vi "earthquake and Tsunami version 2.vi"() -> ()   [LabVIEW 2019]
uses:
  <vilib>/imath/engines/lvmath2/RunTimeEngine/Managers/WorkSpace/UID Generator.vi
  <vilib>/imath/engines/lvmath2/RunTimeEngine/RunTimeType/NIMS_RunTimeType_From StrictType (excl LVString).vi
  <instcachedir>/0/NIMS_RunTimeType_From StrictType (excl LVString)_6DA94F09978249AAA8963F8D3C6FF051.lvgen/NIMS_RunTimeType_From StrictType (excl LVString)_6DA94F09978249AAA8963F8D3C6FF051_000.vi
  <vilib>/imath/engines/lvmath2/RunTimeEngine/LocalVariableDefStatement/MC_LocalVariableDefStatement_Display.vi
  <vilib>/imath/engines/lvmath2/RunTimeEngine/Managers/SymbolTable/Clear UID.vi
  <vilib>/imath/engines/lvmath2/RunTimeEngine/NodeEndStatement/NIMS_NodeEndStatement_Output.vi
  <instcachedir>/0/NIMS_NodeEndStatement_Output_53EC0D466D134D7ABD903AC30B43404B.lvgen/NIMS_NodeEndStatement_Output_53EC0D466D134D7ABD903AC30B43404B_001.vi
  <vilib>/imath/engines/lvmath2/RunTimeEngine/ErrorHandling/NIMS_Finalize Error.vi
  <vilib>/imath/engines/lvmath2/RunTimeEngine/Managers/SymbolTable/NIMS_WorkSpace.lvlib
panel:
  out "Richter Scale Meter":dbl(knob) scale=0.0..10.0
  out "x+y":i32
  out "M (Richter Scale)":dbl
  in  "Amplitude (1*10^-6 m)":dbl
  in  "Distance (1*10^3 m)":dbl
  out "Earthquake":bool
  out "Tsunami":bool
  out "Normal":bool
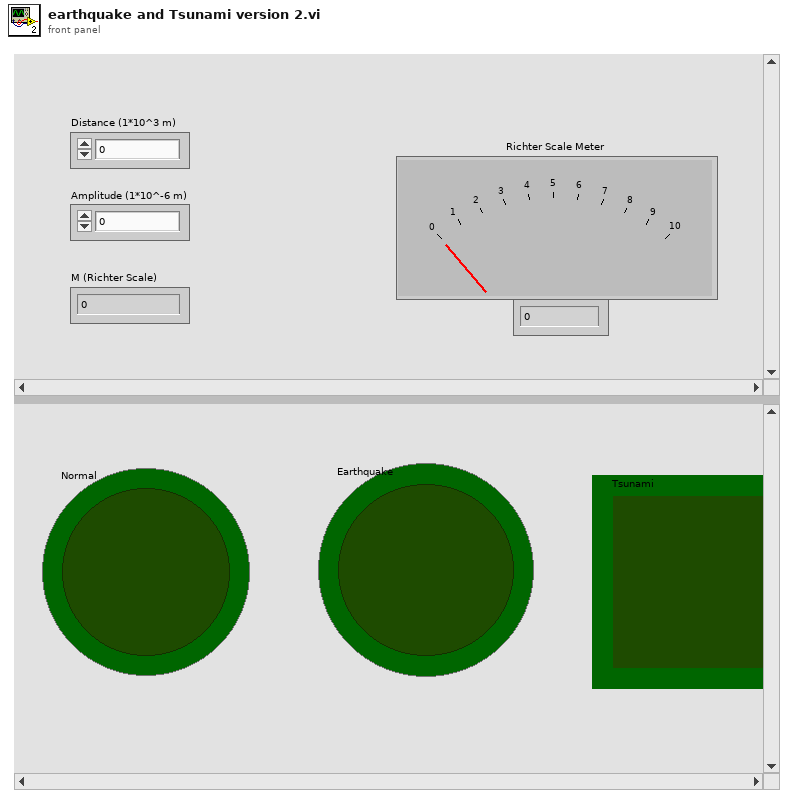
[diagram p1: front panel]
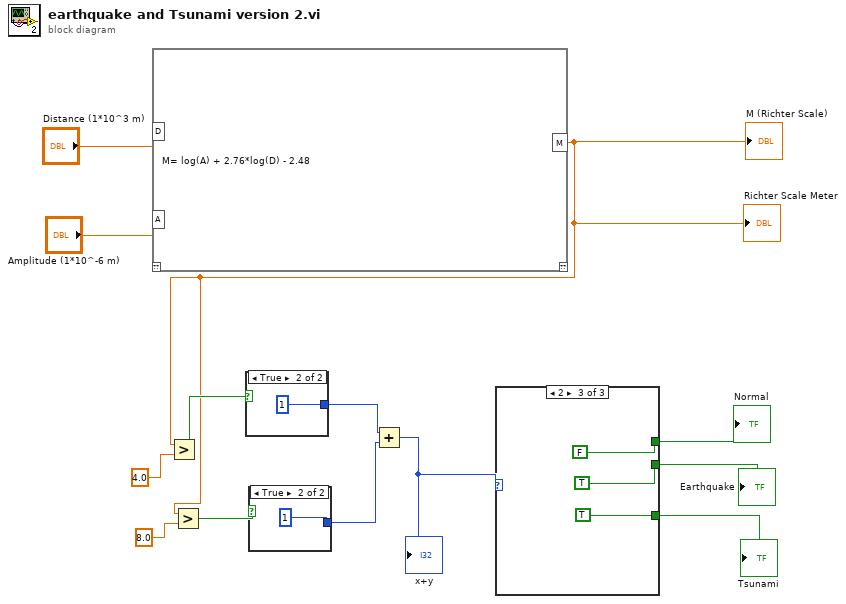
[diagram p0: block diagram]
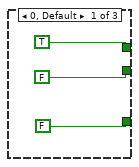
[diagram p2: hidden frame]
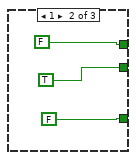
[diagram p3: hidden frame]
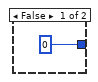
[diagram p4: hidden frame]
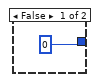
[diagram p5: hidden frame]
diagram:
  n1 = mathscript code="M= log(A) + 2.76*log(D) - 2.48"("D"="Distance (1*10^3 m)", "A"="Amplitude (1*10^-6 m)") -> ("M"=w1:dbl)  [unwired: 1 in, 1 out]
  "M (Richter Scale)" <- w1
  "Richter Scale Meter" <- w1
  n2 = Greater?(x=w1, y=4.0) -> (0:w9:bool)
  n3 = Greater?(x=w1, y=8.0) -> (0:w8:bool)
  n4 = case shown="True" w9 {
    tunnel: [0 1] -> w7
    frame False {
    }
    frame True {
    }
  }
  n5 = case shown="True" w8 {
    tunnel: [0 1] -> w6
    frame False {
    }
    frame True {
    }
  }
  n6 = Add(x=w7, y=w6) -> (x+y=w5:i32)
  "x+y" <- w5
  n7 = case shown="2" w5 {
    tunnel: [TRUE FALSE FALSE] -> w4
    tunnel: [FALSE TRUE TRUE] -> w3
    tunnel: [FALSE FALSE TRUE] -> w2
    frame 0, Default {
    }
    frame 1 {
    }
    frame 2 {
    }
  }
  "Normal" <- w4
  "Tsunami" <- w2
  "Earthquake" <- w3
